vi "Untitled 3.vi"() -> ()   [LabVIEW 2025]
uses:
  <vilib>/Instr/_visa.llb/VISA Configure Serial Port (Instr).vi
panel:
  in  "String 2":string
  in  "Boolean":bool
  out "error out":errorcluster
  out "Meter":dbl(knob) scale=0.0..5.0 scale format="%#_6f"
  out "Numeric":dbl
  out "String":string
  in  "VISA resource name":refnum<visa-resource-name>
  in  "stop":bool
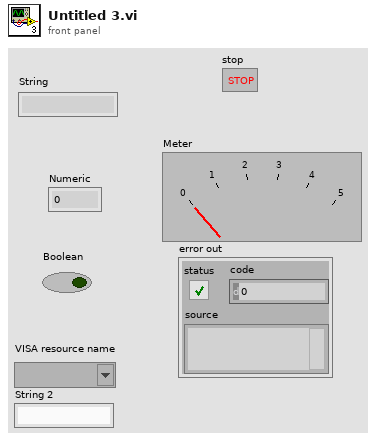
[diagram p1: front panel]
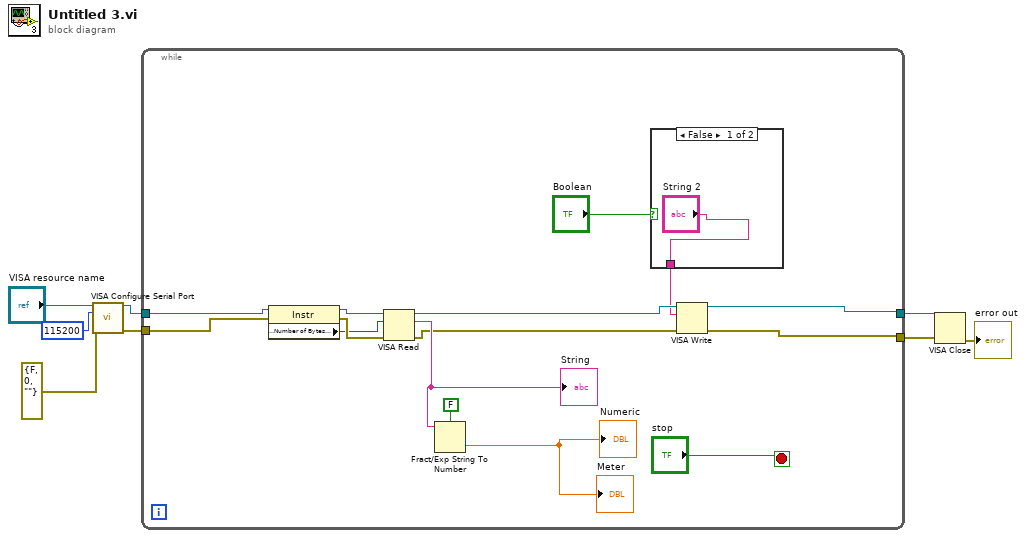
[diagram p0: block diagram]
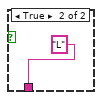
[diagram p2: hidden frame]
diagram:
  n1 = call-poly "VISA Configure Serial Port"("VISA resource name"="VISA resource name", "baud rate (9600)"=u32 115200, "error in (no error)"=errorcluster {"status"=FALSE, "code"=0, "source"=""}) -> ("VISA resource name out"=w8:refnum<visa-resource-name>, "error out"=w6:errorcluster)  [unwired: 11 in]
  n2 = while {
    tunnel: w8 -> [w22]
    tunnel: [w10] -> w7
    tunnel: w6 -> [w20]
    tunnel: [w9] -> w5
    stop <- "stop" stop-if-true
    n3 = property class="Instr"(reference=w22, error in=w20) -> (reference out=w21:refnum<visa-resource-name>, error out=w19:errorcluster, "Serial Settings:Number of Bytes at Serial Port"=w18:u32)
    n4 = VISA Read(VISA resource name=w21, byte count=w18, error in (no error)=w19) -> (VISA resource name out=w14:refnum<visa-resource-name>, read buffer=w17:string, error out=w13:errorcluster)  [unwired: 1 out]
    "String" <- w17
    n5 = Fract/Exp String To Number(use system decimal point (T)=FALSE, string=w17) -> (number=→"Numeric" →"Meter":dbl)  [unwired: 2 in, 1 out]
    n6 = case shown="False" "Boolean" {
      tunnel: ["String 2" "L"] -> w11
      frame False {
      }
      frame True {
      }
    }
    n7 = VISA Write(VISA resource name=w14, write buffer=w11, error in (no error)=w13) -> (VISA resource name out=w10:refnum<visa-resource-name>, error out=w9:errorcluster)  [unwired: 1 out]
  }
  n8 = VISA Close(VISA resource name=w7, error in (no error)=w5) -> (error out=→"error out":errorcluster)
